vi "08_LOGfilewrite.vi"(6 "DAC1cur":dbl, 8 "Regression":cluster{"ResVoltage, V":dbl, "Field, kV/cm":dbl}, 9 "Counters":T1, 10 "Input ChVoltage":T2, 11 "refnum out":refnum<file>) -> ()   [LabVIEW 2017]
uses:
  <vilib>/Utility/error.llb/whitespace.ctl
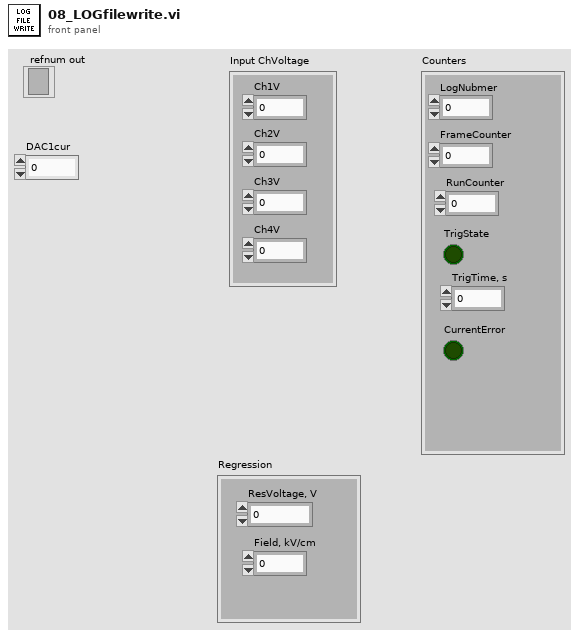
[diagram p1: front panel]
types:
  T1 = cluster{"LogNubmer":i32, "FrameCounter":i32, "RunCounter":u32, "TrigState":bool, "TrigTime, s":dbl, "CurrentError":bool}
  T2 = cluster{"Ch1V":dbl, "Ch2V":dbl, "Ch3V":dbl, "Ch4V":dbl}
  T3 = typedef "whitespace.ctl" = u16
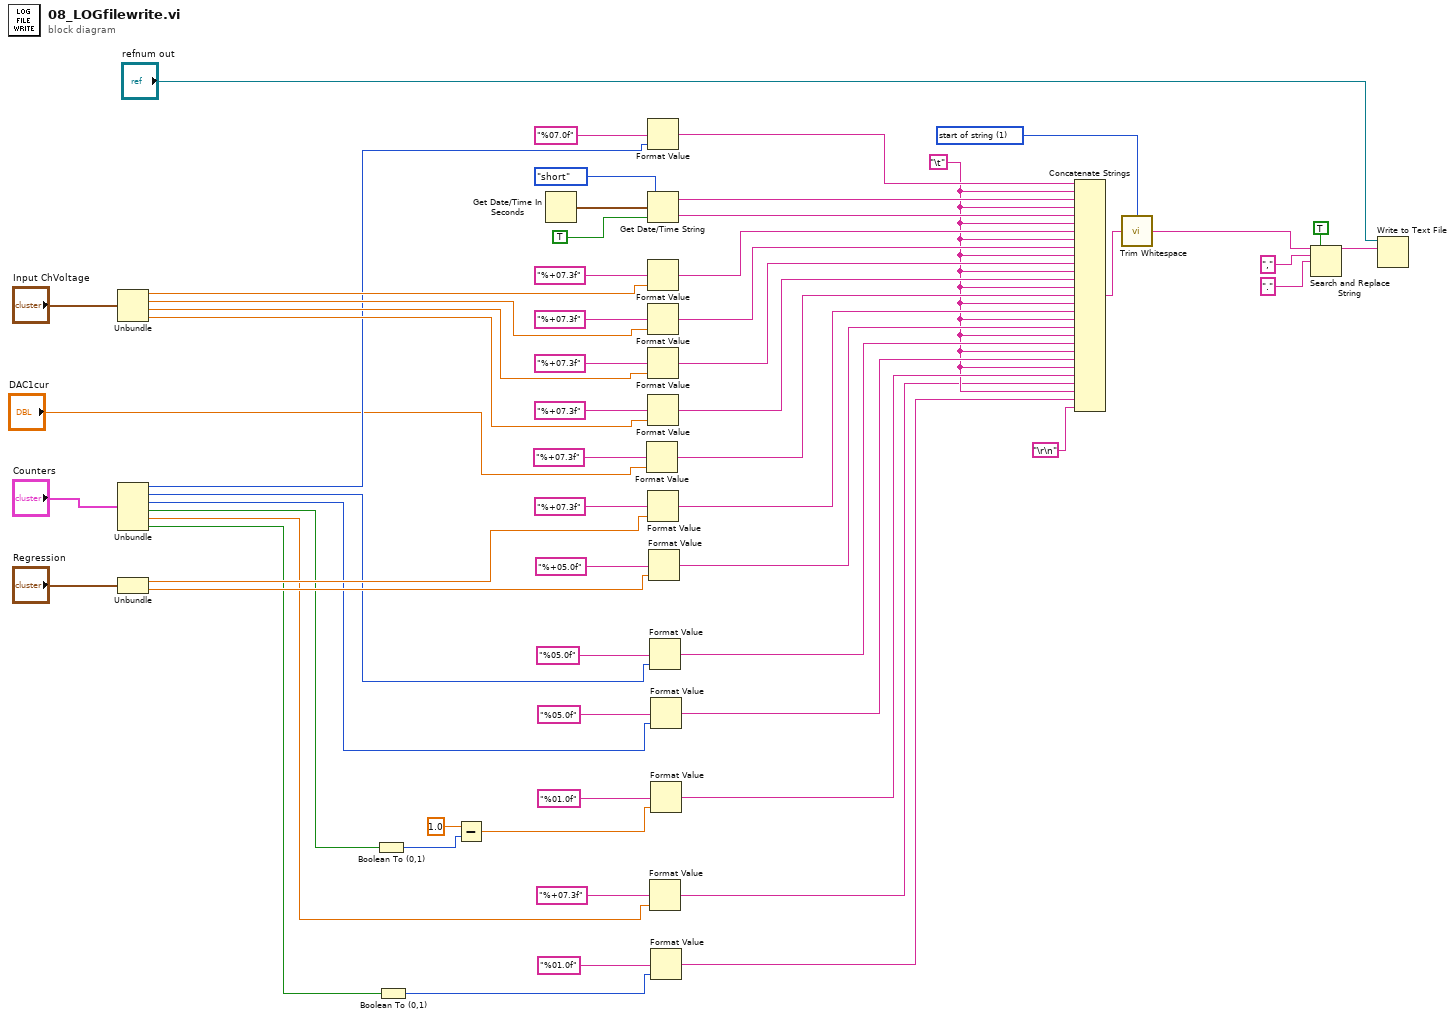
[diagram p0: block diagram]
diagram:
  w9 = "\t"
  w50 = T3 1 items=["both", "start of string", "end of string"] ("location (both)")
  n1 = Unbundle("Input ChVoltage") -> ("Ch1V"=w35:dbl, "Ch2V"=w34:dbl, "Ch3V"=w33:dbl, "Ch4V"=w32:dbl)
  n2 = Unbundle("Counters") -> ("LogNubmer"=w25:i32, "FrameCounter"=w24:i32, "RunCounter"=w23:u32, "TrigState"=w3:bool, "TrigTime, s"=w10:dbl, "CurrentError"=w2:bool)
  n3 = Unbundle("Regression") -> ("ResVoltage, V"=w27:dbl, "Field, kV/cm"=w26:dbl)
  n4 = Boolean To (0,1)(Boolean=w3) -> (0, 1=w4:i16)
  n5 = Boolean To (0,1)(Boolean=w2) -> (0, 1=w1:i16)
  n6 = Subtract(x=1.0, y=w4) -> (x-y=w20:dbl)
  n7 = Get Date/Time In Seconds() -> (seconds since 1Jan1904=w57:timestamp)
  n8 = Format Value(format string="%+07.3f", value (0)="DAC1cur") -> (output string=w13:string)  [unwired: 1 in]
  n9 = Format Value(format string="%07.0f", value (0)=w25) -> (output string=w47:string)  [unwired: 1 in]
  n10 = Get Date/Time String(date format (0)=enum16{"short", "long", "abbreviated"}."short", seconds (now)=w57, want seconds? (F)=TRUE) -> (date string=w48:string, time string=w49:string)
  n11 = Format Value(format string="%+07.3f", value (0)=w35) -> (output string=w54:string)  [unwired: 1 in]
  n12 = Format Value(format string="%+07.3f", value (0)=w34) -> (output string=w53:string)  [unwired: 1 in]
  n13 = Format Value(format string="%+07.3f", value (0)=w33) -> (output string=w52:string)  [unwired: 1 in]
  n14 = Format Value(format string="%+07.3f", value (0)=w32) -> (output string=w40:string)  [unwired: 1 in]
  n15 = Format Value(format string="%+07.3f", value (0)=w27) -> (output string=w14:string)  [unwired: 1 in]
  n16 = Format Value(format string="%+05.0f", value (0)=w26) -> (output string=w15:string)  [unwired: 1 in]
  n17 = Format Value(format string="%05.0f", value (0)=w24) -> (output string=w16:string)  [unwired: 1 in]
  n18 = Format Value(format string="%+07.3f", value (0)=w10) -> (output string=w7:string)  [unwired: 1 in]
  n19 = Format Value(format string="%05.0f", value (0)=w23) -> (output string=w17:string)  [unwired: 1 in]
  n20 = Format Value(format string="%01.0f", value (0)=w20) -> (output string=w18:string)  [unwired: 1 in]
  n21 = Format Value(format string="%01.0f", value (0)=w1) -> (output string=w5:string)  [unwired: 1 in]
  n22 = Concatenate Strings(w47, w9, w48, w9, w49, w9, w54, w9, w53, w9, w52, w9, w40, w9, w13, w9, w14, w9, w15, w9, w16, w9, w17, w9, w18, w7, w9, w5, "\r\n") -> (w51:string)
  n23 = call <vilib>:"Trim Whitespace.vi"("string"=w51, "location (both)"=w50) -> ("trimmed string"=w43:string)
  n24 = Search and Replace String(replace all?=TRUE ("replace all? (F)"), input string=w43, search string=",", replace string="." ("replace string (\"\")")) -> (result string=w42:string)  [unwired: 4 in, 3 out]
  n25 = Write to Text File(file (use dialog)="refnum out", text=w42) -> ()  [unwired: 2 in, 3 out]
